vi "Get System Error.vi"(8 "error in (no error)":errorcluster {"code" format="%.0x"}, 10 "Get Code Cnt":u8, 11 "Device ID (0)":i32) -> (0 "error out":errorcluster {"code" format="%.0x"}, 1 "Error Cnt":u8, 2 "Error Code":u16[](array[numeric]) format="%04x", 3 "Device ID out":i32)   [LabVIEW 2020, in "KEYENCE LJ-X8000A.lvlib"]
doc: "This function gets the controller's system error information.\n\n<B>Note</B>:\nFor the details of the meanings of the error codes that are returned, refer to the \"LJ-X8000A User's Manual\"."
uses:
  KEYENCE LJ-X8000A.lvlib
panel:
  # "(c) 2019 KEYENCE CORPORATION.  ALL RIGHTS RESERVED."
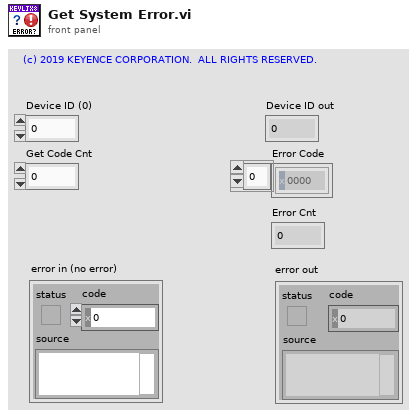
[diagram p1: front panel]
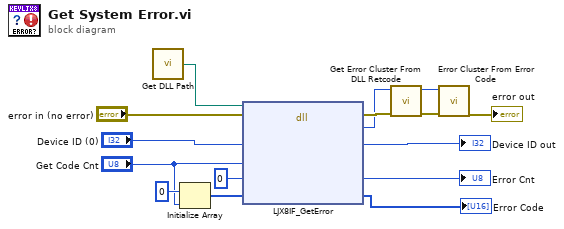
[diagram p0: block diagram]
diagram:
  n1 = call "Get DLL Path.vi"() -> ("DLL Path"=w12:path)  [unwired: 3 in]
  n2 = Initialize Array(u16 0, "Get Code Cnt") -> (w4:u16[])
  n3 = dll-call lib="C:/Program Files (x86)/National Instruments/LabVIEW 2018/instr.lib/KEYENCE LJ-X8000/LJX8_IF.*" fn="LJX8IF_GetError"(path in=w12, error in="error in (no error)", "lDeviceId"="Device ID (0)", "byReceiveMax"="Get Code Cnt", "pbyErrCount"=u8 0 ("pbyErrCnt"), "pwErrCode"=w4) -> (error out=w10:errorcluster, "lRetCode"=w9:i32, "lDeviceId"=→"Device ID out":i32, "pbyErrCount"=→"Error Cnt":u8, "pwErrCode"=→"Error Code":u16[])  [unwired: 2 in, 1 out]
  n4 = call "Get Error Cluster From DLL Retcode.vi"("error in (no error)"=w10, "DLL Return Code"=w9) -> ("error out"=w11:errorcluster, "VI Error Code"=w1:i32)  [unwired: 8 in]
  n5 = call <vilib>:"Error Cluster From Error Code.vi"("error in (no error)"=w11, "error code (0)"=w1) -> ("error out"=→"error out":errorcluster)  [unwired: 7 in]
